vi "Proceso.vi"() -> ()   [LabVIEW 2019, in "Class 2.lvclass"]
uses:
  Class 2.lvclass
  Class 2.lvclass/Class 2.ctl
panel:
  in  "Timer.Timer enable":bool
  in  "Timer.Tiempo deseado":dbl format="%#_13g"
  out "Timer.Timer DN":bool
  in  "stop":bool
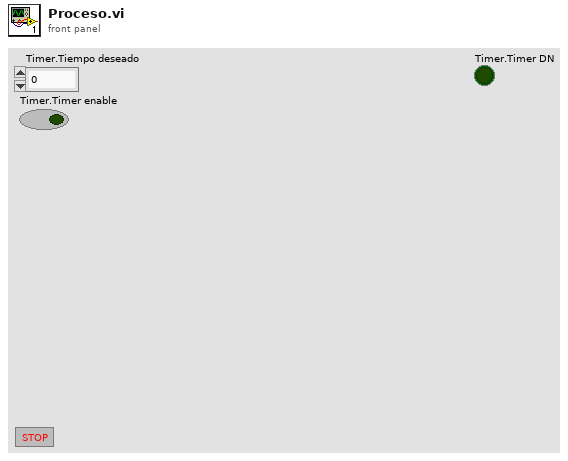
[diagram p1: front panel]
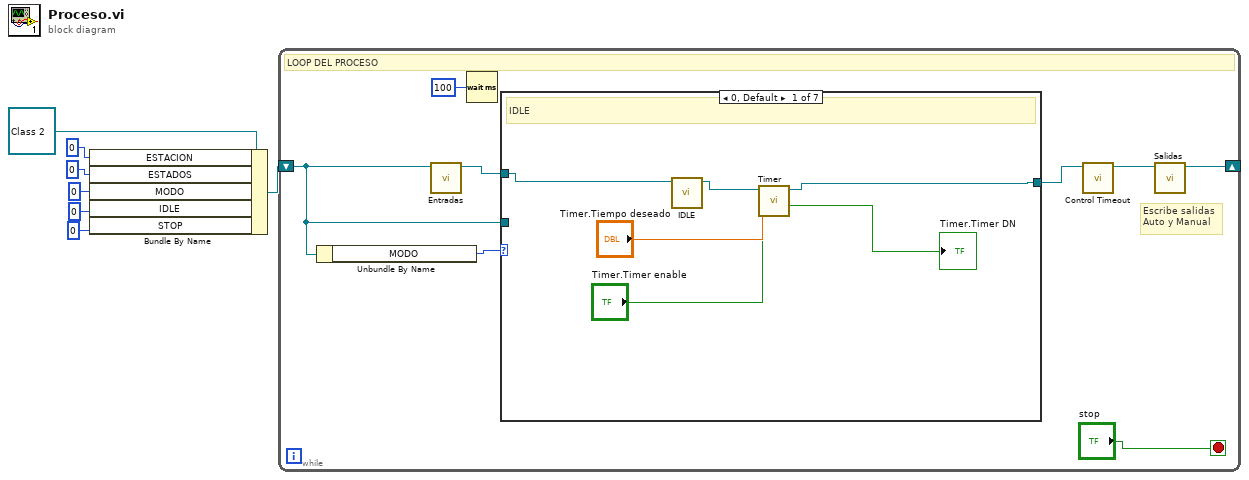
[diagram p0: block diagram]
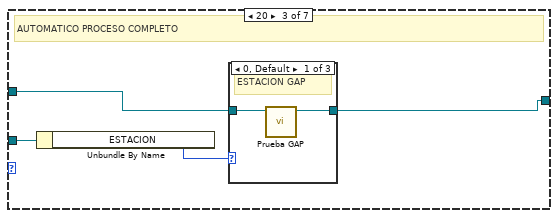
[diagram p3: hidden frame]
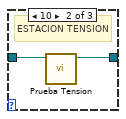
[diagram p4: hidden frame]
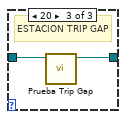
[diagram p5: hidden frame]
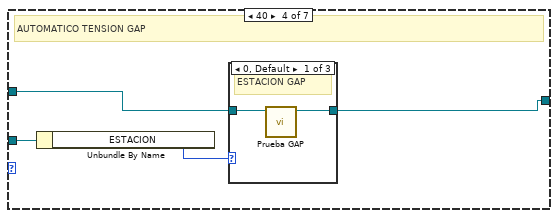
[diagram p6: hidden frame]
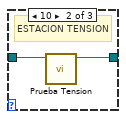
[diagram p7: hidden frame]
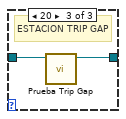
[diagram p8: hidden frame]
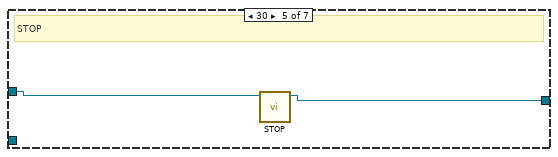
[diagram p9: hidden frame]
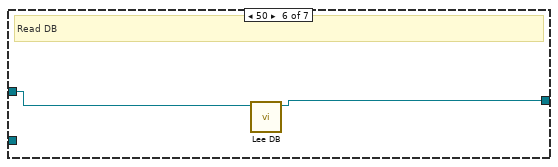
[diagram p10: hidden frame]
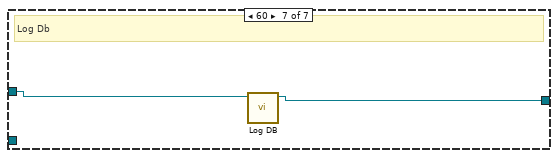
[diagram p11: hidden frame]
diagram:
  n1 = Bundle By Name(cluster=refnum<class "Class 2.lvclass"> refnum ("Class 2.lvclass"), "ESTACION"=0 ("State"), "ESTADOS"=i16 0 ("SubState"), "MODO"=i16 0 ("MAQ DE ESTADOS.MODO"), "IDLE"=i16 0 ("MAQ DE ESTADOS.IDLE"), "STOP"=i16 0 ("MAQ DE ESTADOS.STOP")) -> (w4:refnum<class "Class 2.lvclass">)
  n2 = while {
    shift-right: [w13] -> _
    shift-left: w4 -> [w12]
    stop <- "stop" stop-if-true
    # "Escribe salidas\nAuto y Manual"
    # "LOOP DEL PROCESO"
    n3 = Unbundle By Name(w12) -> ("MODO"=w10:i16)
    n4 = call "Entradas.vi"("Class 2.lvclass"=w12) -> ("Class 2.lvclass 2"=w14:refnum<class "Class 2.lvclass">)  [unwired: 10 in]
    n5 = Wait (ms)(milliseconds to wait=u32 100) -> ()  [unwired: 1 out]
    n6 = case shown="0, Default" w10 {
      tunnel: w12 -> [_ _ w25 w35 _ _ _]
      tunnel: w14 -> [w21 w22 w24 w34 w44 w46 w48]
      tunnel: [w19 w22 w23 w33 w43 w45 w47] -> w9
      frame 0, Default {
        # "IDLE"
        n7 = call "IDLE.vi"("Class 2.lvclass"=w21) -> ("Class 2.lvclass 2"=w20:refnum<class "Class 2.lvclass">)  [unwired: 10 in]
        n8 = call "Timer.vi"("Timer.Timer enable"="Timer.Timer enable", "Timer.Tiempo deseado"="Timer.Tiempo deseado", "Class 2.lvclass"=w20) -> ("Timer.Timer DN"=→"Timer.Timer DN":bool, "Class 2.lvclass 2"=w19:refnum<class "Class 2.lvclass">)  [unwired: 6 in, 1 out]
      }
      frame 10 {
        # "LOGGING"
      }
      frame 20 {
        # "AUTOMATICO PROCESO COMPLETO"
        n9 = Unbundle By Name(w25) -> ("ESTACION"=w26:i32)
        n10 = case shown="0, Default" w26 {
          tunnel: w24 -> [w28 w30 w32]
          tunnel: [w27 w29 w31] -> w23
          frame 0, Default {
            # "ESTACION GAP"
            n11 = call "Prueba GAP.vi"("Class 2.lvclass"=w28) -> ("Class 2.lvclass 2"=w27:refnum<class "Class 2.lvclass">)  [unwired: 10 in]
          }
          frame 10 {
            # "ESTACION TENSION"
            n12 = call "Prueba Tension.vi"("Class 2.lvclass"=w30) -> ("Class 2.lvclass 2"=w29:refnum<class "Class 2.lvclass">)  [unwired: 10 in]
          }
          frame 20 {
            # "ESTACION TRIP GAP"
            n13 = call "Prueba Trip Gap.vi"("Class 2.lvclass"=w32) -> ("Class 2.lvclass 2"=w31:refnum<class "Class 2.lvclass">)  [unwired: 10 in]
          }
        }
      }
      frame 40 {
        # "AUTOMATICO TENSION GAP"
        n14 = Unbundle By Name(w35) -> ("ESTACION"=w36:i32)
        n15 = case shown="0, Default" w36 {
          tunnel: w34 -> [w38 w40 w42]
          tunnel: [w37 w39 w41] -> w33
          frame 0, Default {
            # "ESTACION GAP"
            n16 = call "Prueba GAP.vi"("Class 2.lvclass"=w38) -> ("Class 2.lvclass 2"=w37:refnum<class "Class 2.lvclass">)  [unwired: 10 in]
          }
          frame 10 {
            # "ESTACION TENSION"
            n17 = call "Prueba Tension.vi"("Class 2.lvclass"=w40) -> ("Class 2.lvclass 2"=w39:refnum<class "Class 2.lvclass">)  [unwired: 10 in]
          }
          frame 20 {
            # "ESTACION TRIP GAP"
            n18 = call "Prueba Trip Gap.vi"("Class 2.lvclass"=w42) -> ("Class 2.lvclass 2"=w41:refnum<class "Class 2.lvclass">)  [unwired: 10 in]
          }
        }
      }
      frame 30 {
        # "STOP"
        n19 = call "STOP.vi"("Class 2.lvclass"=w44) -> ("Class 2.lvclass 2"=w43:refnum<class "Class 2.lvclass">)  [unwired: 10 in]
      }
      frame 50 {
        # "Read DB"
        n20 = call "Lee DB.vi"("Class 2 in"=w46) -> ("Class 2 out"=w45:refnum<class "Class 2.lvclass">)  [unwired: 9 in, 1 out]
      }
      frame 60 {
        # "Log Db"
        n21 = call "Log DB.vi"("Class 2 in"=w48) -> ("Class 2 out"=w47:refnum<class "Class 2.lvclass">)  [unwired: 9 in, 1 out]
      }
    }
    n22 = call "Control Timeout.vi"("Class 2 in"=w9) -> ("Class 2 out"=w8:refnum<class "Class 2.lvclass">)  [unwired: 10 in]
    n23 = call "Salidas.vi"("Class 2.lvclass"=w8) -> ("Class 2.lvclass 2"=w13:refnum<class "Class 2.lvclass">)  [unwired: 10 in]
  }
